vi "Configure Data Log Trigger Source.vi"(8 "error in (no error)":errorcluster {"code" format="%.0x"}, 9 "Data Log Trigger Source (2: Immediate)":i32(ring)=2 items=["External", "Software", "Immediate", "Voltage1", "Voltage2", "Voltage3", "Voltage4", "Current1", "Current2", "Current3", "Current4"], 11 "VISA resource name":refnum<visa-resource-name>) -> (0 "error out":errorcluster {"code" format="%.0x"}, 3 "VISA resource name out":refnum<visa-resource-name>)   [LabVIEW 2016, in "Agilent N6700 Series.lvlib"]
doc: "Configures the trigger source of the data logger. When the power supply receives a trigger signal on the source you specify, it runs the data logger.\n\n<b>Note:</b>\nThis VI only applies to the N6705B and N6705C DC Power Analyzer."
uses:
  <instrlib>/Agilent N6700 Series/Agilent N6700 Series.lvlib
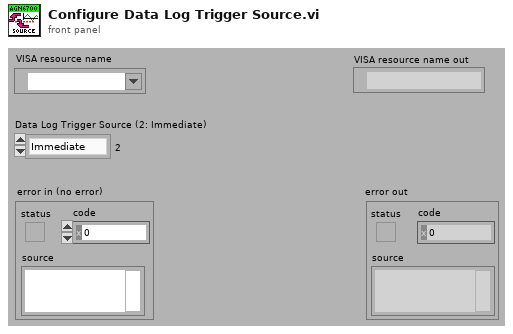
[diagram p1: front panel]
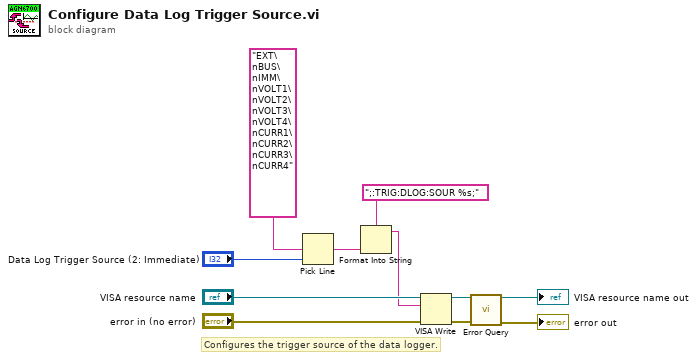
[diagram p0: block diagram]
diagram:
  # "Configures the trigger source of the data logger."
  n1 = Pick Line(multi-line string="EXT\nBUS\nIMM\nVOLT1\nVOLT2\nVOLT3\nVOLT4\nCURR1\nCURR2\nCURR3\nCURR4", line index="Data Log Trigger Source (2: Immediate)") -> (output string=w2:string)  [unwired: 1 in]
  n2 = Format Into String(format string=";:TRIG:DLOG:SOUR %s;", w2) -> (resulting string=w1:string)  [unwired: 2 in, 1 out]
  n3 = VISA Write(VISA resource name="VISA resource name", write buffer=w1, error in (no error)="error in (no error)") -> (VISA resource name out=w7:refnum<visa-resource-name>, error out=w6:errorcluster)  [unwired: 1 out]
  n4 = call <instrlib>:"Error Query.vi"("VISA resource name"=w7, "error in (no error)"=w6) -> ("VISA resource name out"=→"VISA resource name out":refnum<visa-resource-name>, "error out"=→"error out":errorcluster)  [unwired: 10 in, 2 out]
